vi "Add To Drink.vi"(10 "Abstract Beverage":refnum<class "Abstract Beverage.lvclass">, 11 "Condiment Decorator in":refnum<class "Condiment Decorator.lvclass">) -> (3 "Condiment Decorator out":refnum<class "Condiment Decorator.lvclass">)   [LabVIEW 2013, in "Condiment Decorator.lvclass"]
uses:
  Condiment Decorator.lvclass
  Abstract Beverage/Abstract Beverage.lvclass
  Condiment Decorator.lvclass/Condiment Decorator.ctl
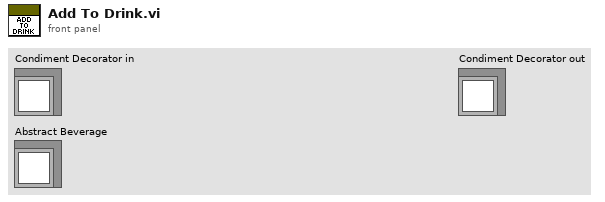
[diagram p1: front panel]
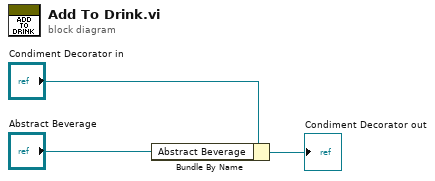
[diagram p0: block diagram]
diagram:
  n1 = Bundle By Name(cluster="Condiment Decorator in", "Abstract Beverage"="Abstract Beverage") -> (→"Condiment Decorator out":refnum<class "Condiment Decorator.lvclass">)
